vi "Init Lidar Labview.vi"(8 "error in (no error)":errorcluster) -> (0 "error out":errorcluster)   [LabVIEW 2018]
uses:
  <instrlib>/Hokuyo URG Series/Public/Initialize-Standard.vi
  control/Control Globals.vi
  Lidar Globals.vi
  <instrlib>/Hokuyo URG Series/Hokuyo URG Series.lvlib
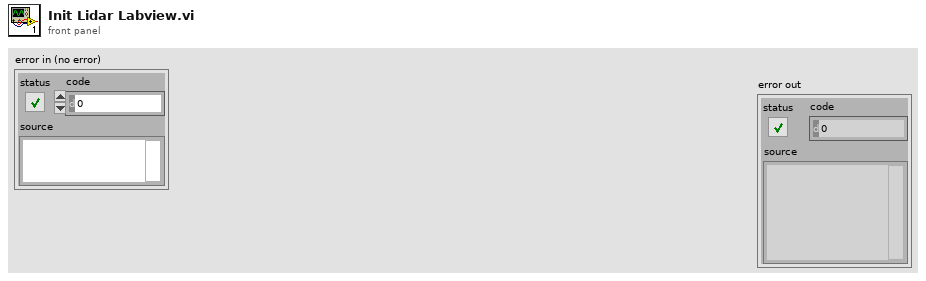
[diagram p1: front panel]
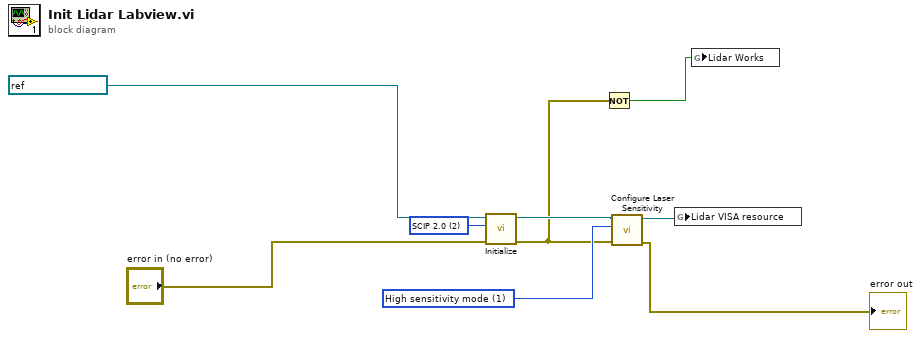
[diagram p0: block diagram]
diagram:
  w5 = u32 1 items=["Normal mode", "High sensitivity mode"] ("Sensitivity Mode (0: Normal mode)")
  w8 = u32 2 items=["Convert to Latest", "SCIP 1.1", "SCIP 2.0"] ("Protocol (2: SCIP 2.0)")
  n1 = call-poly <instrlib>:"Initialize.vi"("error in (no error)"="error in (no error)", "Protocol (2: SCIP 2.0)"=w8, "VISA resource name"=refnum<visa-resource-name> "ASRL3::INSTR") -> ("error out"=w1:errorcluster, "VISA resource name out"=w6:refnum<visa-resource-name>)  [unwired: 7 in]
  n2 = Not(x=w1) -> (.not. x?=w2:bool)
  n3 = call <instrlib>:"Configure Laser Sensitivity.vi"("error in (no error)"=w1, "Sensitivity Mode (0: Normal mode)"=w5, "VISA resource name"=w6) -> ("error out"=→"error out":errorcluster, "VISA resource name out"=w3:refnum<visa-resource-name>)  [unwired: 7 in]
  n4 = global write "Lidar Globals.vi" "Lidar VISA resource"(w3) -> ()
  n5 = global write "Control Globals.vi" "Lidar Works"(w2) -> ()
